vi "Compose Cluster - Nested - Element Value.vi"() -> ()   [LabVIEW 2017, in "Composition.Tests.lvlib"]
uses:
  Composition.Tests.lvlib
  f6fc4eb9-e7a7-4852-a813-db0bbdb44d84.vi
  <vilib>/addons/_JKI Toolkits/Caraya/classes/Test/Test.lvclass
  <vilib>/addons/_JKI Toolkits/Caraya/classes/Assert/Assert.lvclass
panel:
  out "error out":errorcluster
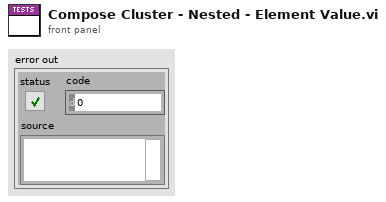
[diagram p1: front panel]
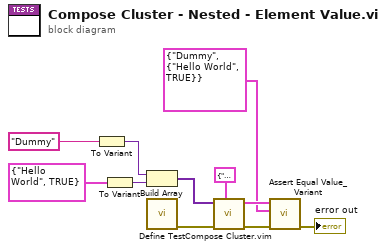
[diagram p0: block diagram]
diagram:
  n1 = To Variant(anything="Dummy") -> (Variant=w7:variant)
  n2 = To Variant(anything=cluster{string, bool} {"Hello World", TRUE}) -> (Variant=w10:variant)
  n3 = Build Array(w7, w10) -> (w9:variant[])
  n4 = call <vilib>:"Define Test.vi"() -> ("error out"=w3:errorcluster)  [unwired: 11 in]
  n5 = call "Compose Cluster.vim"("Type"=cluster{string, cluster{string, bool}} {"", {"", FALSE}}, "error in"=w3, "Elements"=w9) -> ("error out"=w5:errorcluster, "Cluster"=w2:cluster{string, cluster{string, bool}})  [unwired: 7 in]
  n6 = call <vilib>:"Assert Equal Value_Variant.vi"("error in (no error)"=w5, "Y"=cluster{string, cluster{string, bool}} {"Dummy", {"Hello World", TRUE}}, "X"=w2) -> ("error out"=→"error out":errorcluster)  [unwired: 8 in]
